vi "Delimiter.vi"(10 "error in (no error)":errorcluster, 11 "Config Manager in":refnum<class "Config Manager.lvclass">) -> (2 "error out":errorcluster, 3 "Name Separator":string)   [LabVIEW 2020, in "CDM-Config.lvlib" / "Config Manager.lvclass"]
uses:
  Config Manager.lvclass
  Config Manager.lvclass/Config Manager.ctl
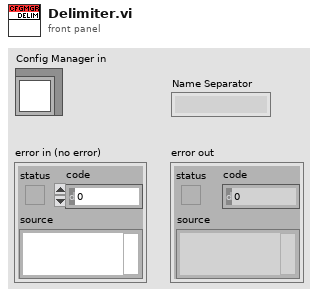
[diagram p1: front panel]
types:
  T1 = typedef "CDM-Config.lvlib/Config Manager.lvclass/Ref Data.ctl" = cluster{"Elements":refnum<class "Config Element.lvclass">[], "Name Separator":string, "Hierarchy Map":map{string[], i32}, "Meta Name Map":map{string, i32[]}}
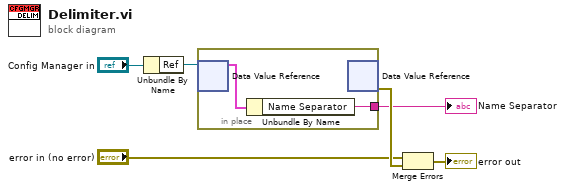
[diagram p0: block diagram]
diagram:
  n1 = Unbundle By Name("Config Manager in") -> ("Ref"=w4:refnum<data-value>)
  n2 = in-place {
    in-place-border: [w7] -> w2
    n3 = in-place-dvr #1(w4) -> (w8:T1)  [unwired: 1 out]
    n4 = Unbundle By Name(w8) -> ("Name Separator"=w7:string)
    n5 = in-place-dvr #1() -> (w6:errorcluster)  [unwired: 1 in, 1 out]
  }
  "Name Separator" <- w2
  n6 = Merge Errors("error in (no error)", w6) -> (→"error out":errorcluster)
